vi "VI Shut Down.vi"(11 "VI Referenz":refnum<vi>) -> ()   [LabVIEW 2020, in "allgemeine Sub-VIs.lvlib"]
uses:
  allgemeine Sub-VIs.lvlib
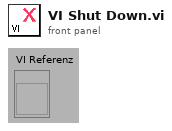
[diagram p1: front panel]
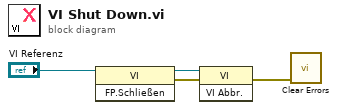
[diagram p0: block diagram]
diagram:
  n1 = invoke class="VI" method="FP.Schließen"(reference="VI Referenz") -> (reference out=w3:refnum<vi>, error out=w2:errorcluster)  [unwired: 2 in, 1 out]
  n2 = invoke class="VI" method="VI Abbr."(reference=w3, error in=w2) -> (error out=w1:errorcluster)  [unwired: 1 in, 2 out]
  n3 = call <vilib>:"Clear Errors.vi"("error in (no error)"=w1) -> ()  [unwired: 5 in, 2 out]
